vi "Visa set timeot and termination.vi"(6 "Termination Character Enable":bool, 7 "Termination Character Enable Based on Interface":bool, 8 "error in (no error)":errorcluster, 9 "Termination Character":u8=10, 10 "Timeout Value":u32, 11 "VISA resource name":refnum<visa-resource-name>) -> (0 "error out":errorcluster, 1 "Old Termination Character":u8=13, 2 "Old Timeout Value":u32, 3 "VISA resource name out":refnum<visa-resource-name>, 4 "Old Termination Character Enable":bool)   [LabVIEW 2023]
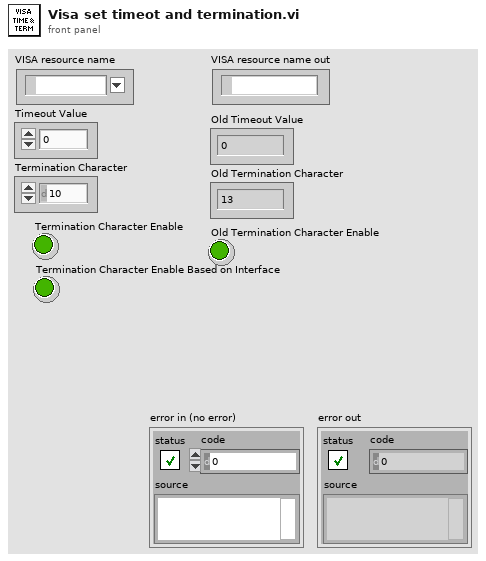
[diagram p1: front panel]
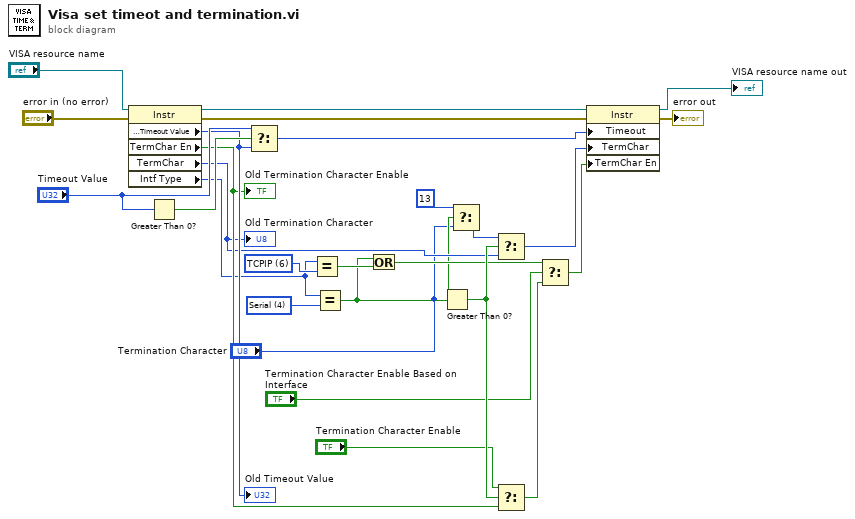
[diagram p0: block diagram]
diagram:
  w7 = u16 4 items=["GPIB"=1, "VXI"=2, "GPIB-VXI"=3, "Serial"=4, "PXI"=5, "TCPIP"=6, "USB"=7, "FireWire"=9] ("Interface Information:Interface Type")
  w12 = u16 6 items=["GPIB"=1, "VXI"=2, "GPIB-VXI"=3, "Serial"=4, "PXI"=5, "TCPIP"=6, "USB"=7, "FireWire"=9] ("Interface Information:Interface Type")
  n1 = property class="Instr"(reference="VISA resource name", error in="error in (no error)") -> (reference out=w26:refnum<visa-resource-name>, error out=w24:errorcluster, "General Settings:Timeout Value"=w19:u32, "TermChar En"=w14:bool, "TermChar"=w13:u8, "Intf Type"=w5:u16)
  "Old Timeout Value" <- w19
  "Old Termination Character" <- w13
  "Old Termination Character Enable" <- w14
  n2 = Greater Than 0?(x="Timeout Value") -> (x > 0?=w21:bool)
  n3 = Select(t="Timeout Value", s=w21, f=w19) -> (s? t:f=w18:u32)
  n4 = Equal?(x=w5, y=w12) -> (x = y?=w10:bool)
  n5 = Equal?(x=w5, y=w7) -> (x = y?=w4:bool)
  n6 = Or(x=w4, y=w10) -> (x .or. y?=w6:bool)
  n7 = Greater Than 0?(x="Termination Character") -> (x > 0?=w16:bool)
  n8 = Select(t=u8 13, s=w4, f="Termination Character") -> (s? t:f=w1:u8)
  n9 = Select(t=w1, s=w16, f=w13) -> (s? t:f=w17:u8)
  n10 = Select(t="Termination Character Enable", s=w16, f=w14) -> (s? t:f=w9:bool)
  n11 = Select(t=w6, s="Termination Character Enable Based on Interface", f=w9) -> (s? t:f=w8:bool)
  n12 = property class="Instr"(reference=w26, error in=w24, "Timeout"=w18, "TermChar"=w17, "TermChar En"=w8) -> (reference out=→"VISA resource name out":refnum<visa-resource-name>, error out=→"error out":errorcluster)
